vi "SubProcess.vi"(7 "Console":refnum<vi>, 8 "error in":errorcluster, 9 "Python version":string="3.9", 11 "Command":string="ping -c 4 python.org") -> (0 "error out":errorcluster, 2 "text":string)   [LabVIEW 2021]
panel:
  out "RETURN CODE":string
  out "return value":string[](array[string])
  out "Array":string[](array[string])
  out "return":string
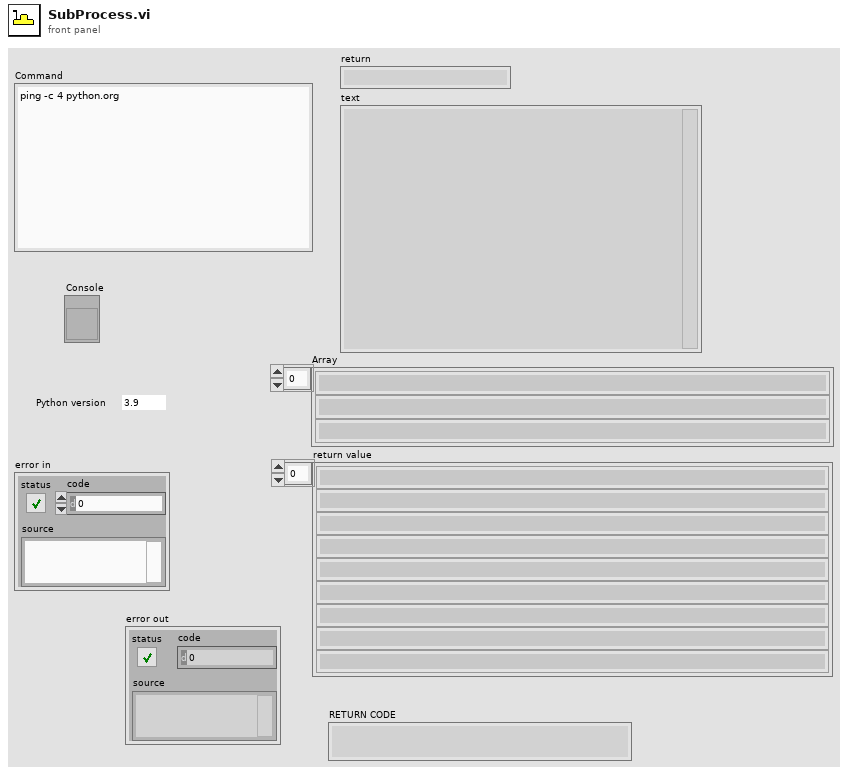
[diagram p1: front panel]
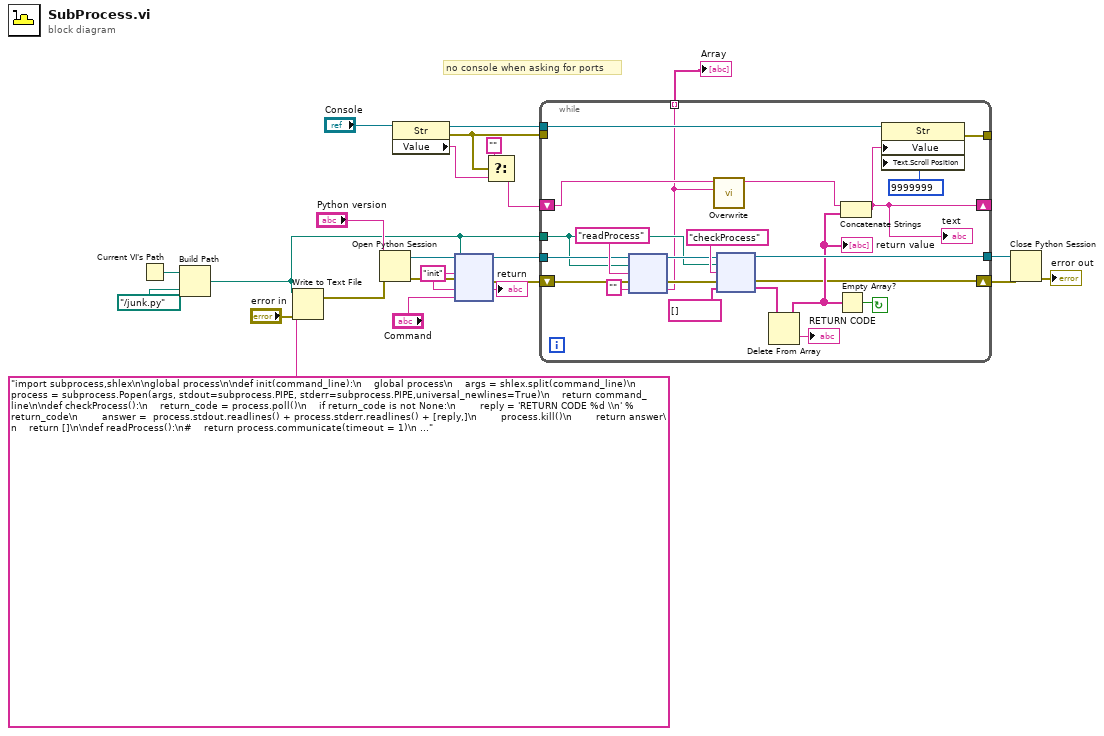
[diagram p0: block diagram]
diagram:
  w21 = "init" ("function name")
  # "no console when asking for ports"
  n1 = Current VI's Path() -> (path=w3:path)
  n2 = Build Path(base path=w3, name or relative path=path "../junk.py" ("file (use dialog)")) -> (appended path=w1:path)
  n3 = Write to Text File(file (use dialog)=w1, text="import subprocess,shlex\n\nglobal process\n\ndef init(command_line):\n    global process\n    args = shlex.split(command_line)\n    process = subprocess.Popen(args, stdout=subprocess.PIPE, stderr=subprocess.PIPE,universal_newlines=True)\n    return command_line\n\ndef checkProcess():\n    return_code = process.poll()\n    if return_code is not None:\n        reply = 'RETURN CODE %d \\n' % return_code\n        answer =  process.stdout.readlines() + process.stderr.readlines() + [reply,]\n        process.kill()\n        return answer\n    return []\n\ndef readProcess():\n#    return process.communicate(timeout = 1)\n    return process.stdout.readline() \n", error in="error in") -> (error out=w22:errorcluster)  [unwired: 1 in, 2 out]
  n4 = Open Python Session(python version="Python version", 3:w22) -> (session out=w23:refnum<k35>, error out=w7:errorcluster)  [unwired: 1 in]
  n5 = property class="Str"(reference="Console") -> (reference out=w16:refnum<vi>, error out=w14:errorcluster, "Value"=w13:string)  [unwired: 1 in]
  n6 = node(w23, w1, w21, w7, w21, "Command") -> (w19:refnum<k35>, w6:errorcluster, →"return":string)  [unwired: 1 in, 2 out]
  n7 = Select(t="" ("function name"), s=w14, f=w13) -> (s? t:f=w12:string)
  n8 = while {
    tunnel: w1 -> [w39]
    tunnel: w19 -> [w45]
    shift-right: [w34] -> _
    shift-left: w12 -> [w32]
    tunnel: [w37] -> w18
    tunnel: w16 -> [w35]
    tunnel: w14 -> [_]
    tunnel: [w33] -> _
    tunnel: [w30] -> w10 mode=indexing
    shift-right: [w25] -> w5
    shift-left: w6 -> [w26]
    stop <- w40 continue-if-true
    n9 = node(w45, w39, "readProcess" ("function name"), w26, "") -> (w43:refnum<k35>, w38:errorcluster, w30:string)  [unwired: 2 out]
    n10 = call "Overwrite.vi"("String"=w30, "Value in"=w32) -> ("Value out"=w31:string)  [unwired: 9 in]
    n11 = node(w43, w39, "checkProcess" ("function name"), w38, string[] []) -> (w37:refnum<k35>, w25:errorcluster, w29:string[])  [unwired: 2 out]
    n12 = Delete From Array(array=w29) -> (deleted portion=→"RETURN CODE":string, array with subset deleted=w28:string[])  [unwired: 2 in]
    "return value" <- w28
    n13 = Empty Array?(array=w28) -> (empty?=w40:bool)
    n14 = Concatenate Strings(w31, w28) -> (w34:string)
    "text" <- w34
    n15 = property class="Str"(reference=w35, "Value"=w34, "Text.Scroll Position"=u32 9999999) -> (error out=w33:errorcluster)  [unwired: 1 in, 1 out]
  }
  "Array" <- w10
  n16 = Close Python Session(session in=w18, error in=w5) -> (11:→"error out":errorcluster)
